vi "HRR-SetID.vi"(10 "ID":u8[](array[numeric])=[0, 0, 0, 0, 0, 0, 0, 0]) -> (0 "error out":errorcluster, 3 "FPGA VI Reference Out":refnum<k20>)   [LabVIEW 2019]
uses:
  <vilib>/FPGAPlugInAG/myRIO-1900/niLvFpga_Open_myRIO-1900.vi
  <vilib>/rvi/interface/common/dynamic/niFpgaDynamicAddResources.vi
  <vilib>/myRIO/Common/Instrument Driver Framework/Utilities/vis/FPGA Ref Manager.vi
  <vilib>/Utility/error.llb/Error Cluster From Error Code.vi
  <vilib>/myRIO/Common/Instrument Driver Framework/Utilities/vis/Ref Counter.vi
  <vilib>/rvi/interface/common/niFpgaWaitOnOcc.vi
  <vilib>/rvi/interface/nirviOpenFPGA/nirviOpenFPGA.xnode
  FPGA Bitfiles/MyRIOFPGATest_FPGATarget_FPGAMainDefault_pJ5Q7Xj1Ujo.lvbitx
  FPGA Main Default.vi
  <vilib>/rvi/interface/nirviMethod/nirviMethod.xnode
  <vilib>/FPGAPlugInAG/Dynamic/niLvFpga_ConfigureFifo_Dynamic.vi
  <vilib>/rvi/errors/niLvFpgaMergeErrorWithErrorCode.vi
  <vilib>/myRIO/Instrument Drivers/Utilities/Utilities.lvlib
panel:
  out "Actual Depth":u32
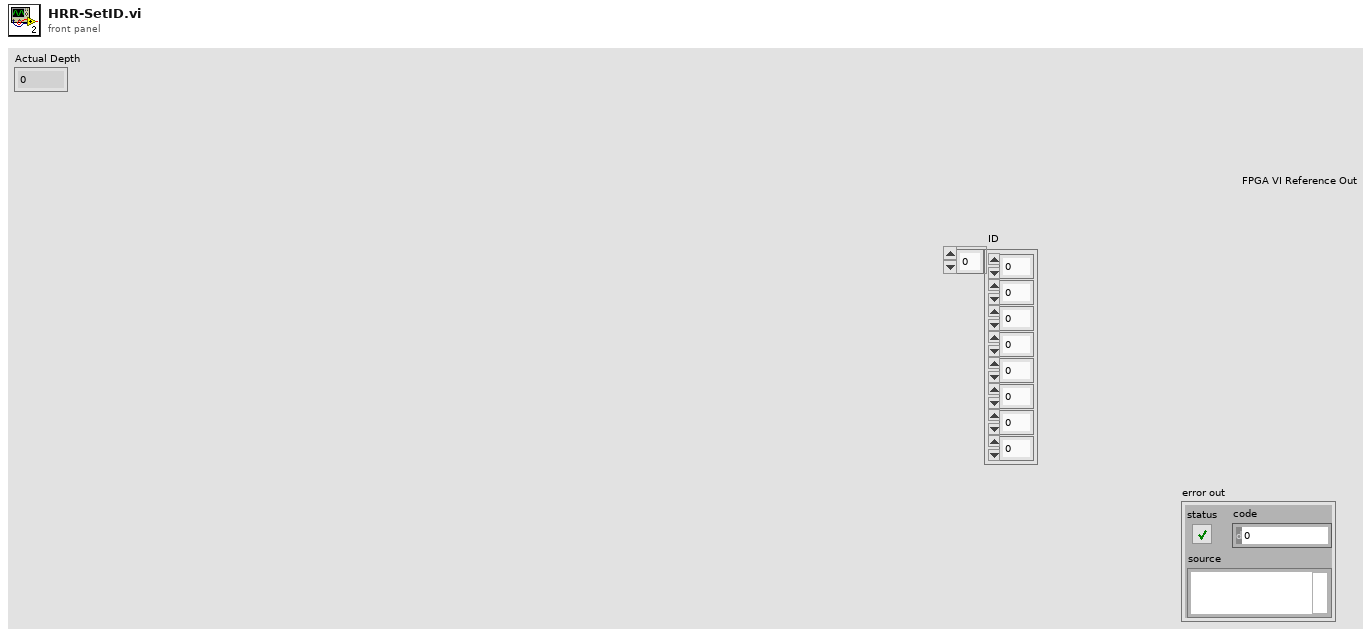
[diagram p1: front panel]
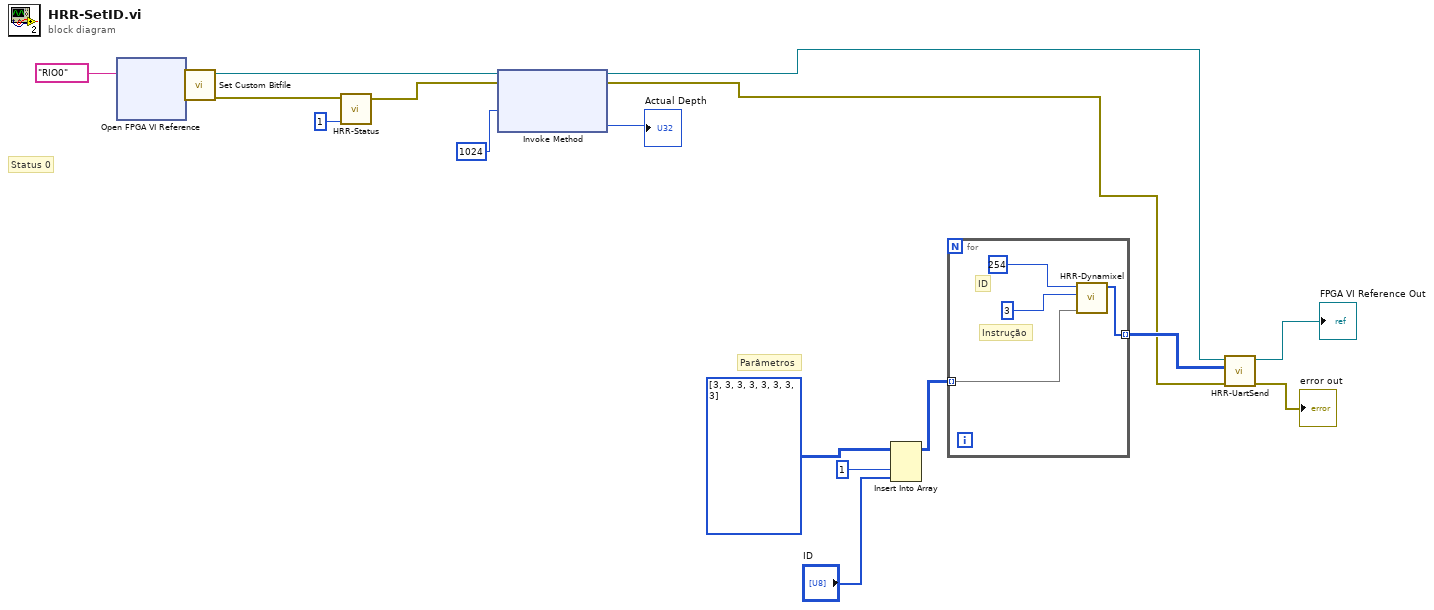
[diagram p0: block diagram]
diagram:
  # "Status 0"
  # "Parâmetros"
  n1 = xnode "Open FPGA VI Reference"("resource name"=tag "RIO0") -> ("FPGA VI Reference Out"=w9:refnum<k20>, "error out"=w10:errorcluster)  [unwired: 1 in]
  n2 = call <vilib>:"Set Custom Bitfile.vi"("error in (no error)"=w10, "Custom FPGA Reference In"=w9) -> ("error out"=w3:errorcluster, "Custom FPGA Reference Out"=w4:refnum<k20>)  [unwired: 8 in]
  n3 = call "HRR-Status.vi"("Status (U4)"=u8 1 ("number"), "error in (no error)"=w3) -> ("error out"=w6:errorcluster)  [unwired: 9 in]
  n4 = xnode "Invoke Method"("FPGA VI Reference In"=w4, "error in"=w6, "Requested Depth"=u32 1024) -> ("FPGA VI Reference Out"=w1:refnum<k20>, "error out"=w2:errorcluster, "Actual Depth"=→"Actual Depth":u32)
  n5 = Insert Into Array(array=u8[][] [[3], [3], [3], [3], [3], [3], [3], [3]], index (col)=1 ("disabled index (col)"), new element="ID") -> (w16:u8[][])  [unwired: 1 in]
  n6 = for {
    tunnel: w16 -> [w20] mode=indexing
    tunnel: [w19] -> w13 mode=indexing
    # "Instrução"
    # "ID"
    n7 = call "HRR-Dynamixel.vi"("ID"=u8 254, "Instruction"=u8 3, "Array in"=w20) -> ("Array out"=w19:u8[])  [unwired: 7 in]
  }
  n8 = call "HRR-UartSend.vi"("error in (no error)"=w2, "Array"=w13, "Refnum in"=w1) -> ("error out"=→"error out":errorcluster, "Refnum out"=→"FPGA VI Reference Out":refnum<k20>)  [unwired: 7 in]
